vi "ASI_change_XY_speed.vi"(2 "error in (no error)":errorcluster, 3 "VISA resource name":refnum<visa-resource-name>="COM7", 4 "speed":dbl) -> (0 "error out":errorcluster)   [LabVIEW 2015]
uses:
  <vilib>/Instr/_visa.llb/VISA Flush IO Buffer Mask.ctl
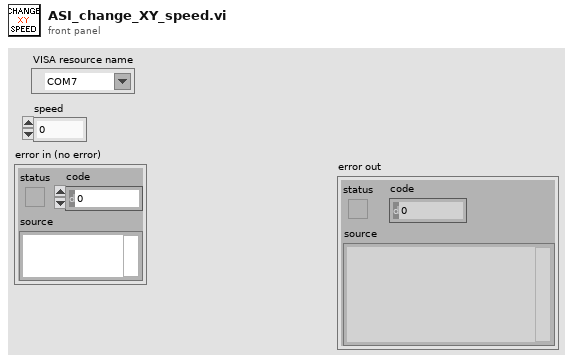
[diagram p1: front panel]
types:
  T1 = typedef "VISA Flush IO Buffer Mask.ctl" = u16
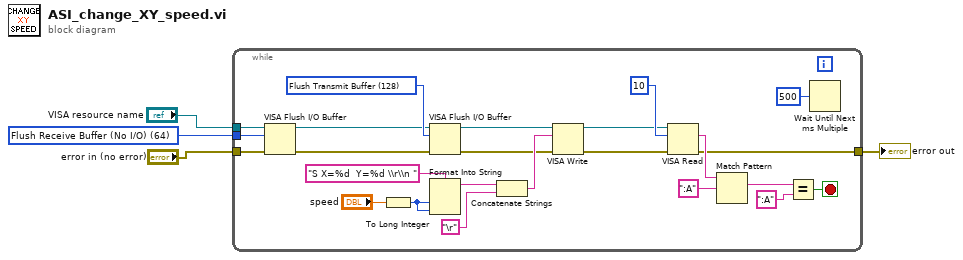
[diagram p0: block diagram]
diagram:
  w3 = T1 64 items=["Flush Receive Buffer"=16, "Write Transmit Buffer to Device"=32, "Flush Receive Buffer (No I/O)"=64, "Flush Transmit Buffer"=128] ("Mask")
  n1 = while {
    tunnel: "error in (no error)" -> [w24]
    tunnel: w3 -> [w18]
    tunnel: "VISA resource name" -> [w17]
    tunnel: [w8] -> w1
    stop <- w7 stop-if-true
    w21 = T1 128 items=["Flush Receive Buffer"=16, "Write Transmit Buffer to Device"=32, "Flush Receive Buffer (No I/O)"=64, "Flush Transmit Buffer"=128] ("Mask")
    n2 = VISA Flush I/O Buffer(VISA resource name=w17, mask (16)=w18, error in (no error)=w24) -> (VISA resource name out=w20:refnum<visa-resource-name>, error out=w19:errorcluster)
    n3 = To Long Integer(number="speed") -> (32bit integer=w15:i32)
    n4 = VISA Flush I/O Buffer(VISA resource name=w20, mask (16)=w21, error in (no error)=w19) -> (VISA resource name out=w23:refnum<visa-resource-name>, error out=w22:errorcluster)
    n5 = Format Into String(format string="S X=%d  Y=%d \\r\\n ", w15, w15) -> (resulting string=w25:string)  [unwired: 2 in, 1 out]
    n6 = Concatenate Strings(w25, "\r") -> (w26:string)
    n7 = VISA Write(VISA resource name=w23, write buffer=w26, error in (no error)=w22) -> (VISA resource name out=w5:refnum<visa-resource-name>, error out=w9:errorcluster)  [unwired: 1 out]
    n8 = VISA Read(VISA resource name=w5, byte count=u32 10, error in (no error)=w9) -> (read buffer=w12:string, error out=w8:errorcluster)  [unwired: 2 out]
    n9 = Match Pattern(string=w12, regular expression=":A" ("y")) -> (match substring=w13:string)  [unwired: 1 in, 3 out]
    n10 = Equal?(x=w13, y=":A") -> (x = y?=w7:bool)
    n11 = Wait Until Next ms Multiple(millisecond multiple=u32 500) -> ()  [unwired: 1 out]
  }
  "error out" <- w1
